vi "Update Properties Clusters in Plugin.vi"(8 "error in":errorcluster, 10 "Channel Types":string[](array[string]), 11 "VI Path":path) -> (0 "error out":errorcluster)   [LabVIEW 2026, in "NIVS_CDEW_MetaDataObj.lvclass"]
uses:
  NIVS_CDEW_MetaDataObj.lvclass
  NIVS_CDEW_MetaDataObj.lvclass/NIVS_CDEW_MetaDataObj.ctl
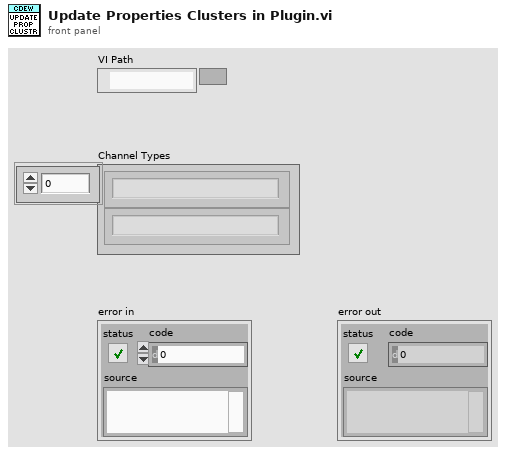
[diagram p1: front panel]
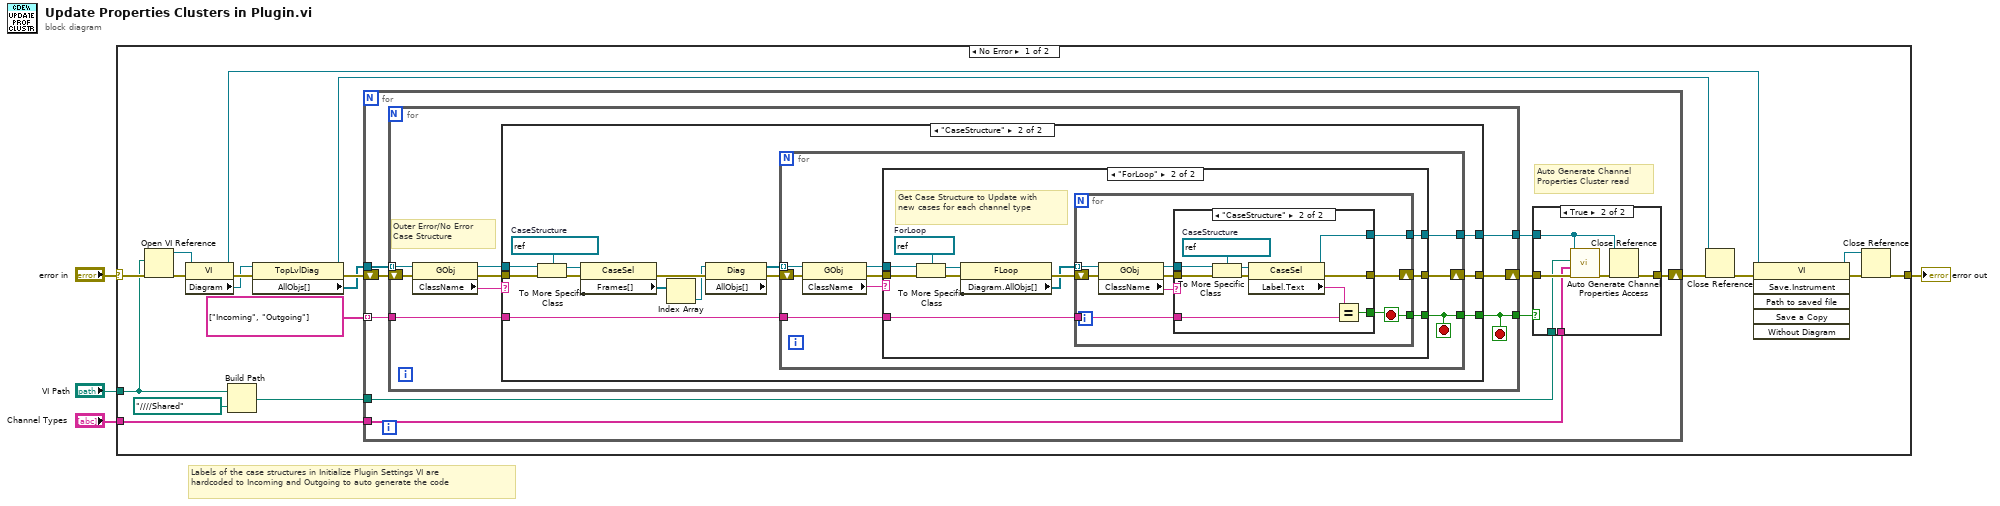
[diagram p0: block diagram]
diagram:
  # "Labels of the case structures in Initialize Plugin Settings VI are\nhardcoded to Incoming and Outgoing to auto generate the code"
  n1 = case shown="No Error" "error in" {
    selector: "error in" -> [w19 w105]
    tunnel: [w17 w105] -> w3
    tunnel: "Channel Types" -> [w10 _]
    tunnel: "VI Path" -> [w5 _]
    frame No Error {
      n2 = Open VI Reference(vi path=w5, error in (no error)=w19) -> (vi reference=w13:refnum<vi>, error out=w21:errorcluster)  [unwired: 4 in]
      n3 = property class="VI"(reference=w13, error in=w21) -> (reference out=w15:refnum<vi>, error out=w20:errorcluster, "Diagram"=w12:refnum<vi>)
      n4 = Build Path(base path=w5, name or relative path=path "../../../../Shared") -> (appended path=w8:path)
      n5 = property class="TopLvlDiag"(reference=w12, error in=w20) -> (reference out=w7:refnum<vi>, error out=w18:errorcluster, "AllObjs[]"=w11:refnum<vi>[])
      n6 = for {
        tunnel: w11 -> [w29]
        tunnel: w10 -> [w27]
        tunnel: w8 -> [w25]
        shift-right: [w30] -> w16
        shift-left: w18 -> [w32]
        tunnel: string[] ["Incoming", "Outgoing"] ("Case Structure Labels") -> [w24] mode=indexing
        # "Auto Generate Channel\nProperties Cluster read"
        n7 = for {
          tunnel: w29 -> [w38] mode=indexing
          tunnel: [w35] -> w28
          tunnel: [w34] -> w26
          shift-right: [w39] -> w31
          shift-left: w32 -> [w41]
          tunnel: w24 -> [w36]
          stop <- w35 stop-if-true
          # "Outer Error/No Error\nCase Structure"
          n8 = property class="GObj"(reference=w38, error in=w41) -> (reference out=w37:refnum<vi>, error out=w40:errorcluster, "ClassName"=w33:string)
          n9 = case shown="\"CaseStructure\"" w33 {
            tunnel: w40 -> [w42 w55]
            tunnel: [w42 w56] -> w39
            tunnel: w37 -> [_ w46]
            tunnel: w36 -> [_ w51]
            tunnel: [_ w50] -> w35
            tunnel: [_ w49] -> w34
            frame Default {
            }
            frame "CaseStructure" {
              w47 = refnum<vi> refnum  # CaseStructure
              n10 = To More Specific Class(target class=w47, reference=w46, error in=w55) -> (specific class reference=w48:refnum<vi>, error out=w54:errorcluster)
              n11 = property class="CaseSel"(reference=w48, error in=w54) -> (error out=w53:errorcluster, "Frames[]"=w45:refnum<vi>[])  [unwired: 1 out]
              n12 = Index Array(array=w45) -> (element=w44:refnum<vi>)  [unwired: 1 in]
              n13 = property class="Diag"(reference=w44, error in=w53) -> (error out=w52:errorcluster, "AllObjs[]"=w43:refnum<vi>[])  [unwired: 1 out]
              n14 = for {
                tunnel: w51 -> [w62]
                tunnel: [w57] -> w50
                tunnel: [w61] -> w49
                shift-right: [w65] -> w56
                shift-left: w52 -> [w64]
                tunnel: w43 -> [w60] mode=indexing
                stop <- w57 stop-if-true
                n15 = property class="GObj"(reference=w60, error in=w64) -> (reference out=w58:refnum<vi>, error out=w63:errorcluster, "ClassName"=w59:string)
                n16 = case shown="\"ForLoop\"" w59 {
                  tunnel: w63 -> [w66 w77]
                  tunnel: [w66 w76] -> w65
                  tunnel: w58 -> [_ w70]
                  tunnel: w62 -> [_ w69]
                  tunnel: [_ w68] -> w57
                  tunnel: [_ w67] -> w61
                  frame Default {
                  }
                  frame "ForLoop" {
                    w72 = refnum<vi> refnum  # ForLoop
                    # "Get Case Structure to Update with new cases for each channel type"
                    n17 = To More Specific Class(target class=w72, reference=w70, error in=w77) -> (specific class reference=w73:refnum<vi>, error out=w75:errorcluster)
                    n18 = property class="FLoop"(reference=w73, error in=w75) -> (error out=w74:errorcluster, "Diagram.AllObjs[]"=w71:refnum<vi>[])  [unwired: 1 out]
                    n19 = for {
                      tunnel: w71 -> [w83] mode=indexing
                      tunnel: w69 -> [w82]
                      tunnel: [w80] -> w68
                      tunnel: [w79] -> w67
                      shift-right: [w86] -> w76
                      shift-left: w74 -> [w84]
                      stop <- w80 stop-if-true
                      n20 = property class="GObj"(reference=w83, error in=w84) -> (reference out=w81:refnum<vi>, error out=w85:errorcluster, "ClassName"=w78:string)
                      n21 = case shown="\"CaseStructure\"" w78 {
                        tunnel: w81 -> [_ w93]
                        tunnel: w82 -> [_ w90]
                        tunnel: [_ w89] -> w80
                        tunnel: w85 -> [w87 w97]
                        tunnel: [w87 w95] -> w86
                        tunnel: [_ w88] -> w79
                        frame Default {
                        }
                        frame "CaseStructure" {
                          w94 = refnum<vi> refnum  # CaseStructure
                          n22 = To More Specific Class(target class=w94, reference=w93, error in=w97) -> (specific class reference=w92:refnum<vi>, error out=w96:errorcluster)
                          n23 = property class="CaseSel"(reference=w92, error in=w96) -> (reference out=w88:refnum<vi>, error out=w95:errorcluster, "Label.Text"=w91:string)
                          n24 = Equal?(x=w91, y=w90) -> (x = y?=w89:bool)
                        }
                      }
                    }
                  }
                }
              }
            }
          }
        }
        n25 = case shown="True" w28 {
          tunnel: w27 -> [_ w99]
          tunnel: [w98 w104] -> w30
          tunnel: w31 -> [w98 w102]
          tunnel: w26 -> [_ w101]
          tunnel: w25 -> [_ w100]
          frame False {
          }
          frame True {
            n26 = call "Auto Generate Channel Properties Access.vi"("error in"=w102, "Channel Types"=w99, "Path"=w100, "Reference in"=w101) -> ("error out"=w103:errorcluster)  [unwired: 7 in]
            n27 = Close Reference(reference=w101, error in (no error)=w103) -> (error out=w104:errorcluster)
          }
        }
      }
      n28 = Close Reference(reference=w7, error in (no error)=w16) -> (error out=w23:errorcluster)
      n29 = invoke class="VI" method="Save.Instrument"(reference=w15, error in=w23) -> (reference out=w14:refnum<vi>, error out=w22:errorcluster)  [unwired: 4 in, 4 out]
      n30 = Close Reference(reference=w14, error in (no error)=w22) -> (error out=w17:errorcluster)
    }
    frame Error {
    }
  }
  "error out" <- w3
